vi "UTILITY Add Newfi Data To List.vi"(6 "Use Default Headers Main":bool, 8 "Error In":errorcluster, 10 "Full Data":string[][](array[string]), 11 "New Header Save Array":T1[](array[typedef])) -> (0 "Error Out":errorcluster, 2 "Data":string[][](array[string]), 3 "Save Data":string[][](array[string]))   [LabVIEW 2016]
uses:
  Washer DOE/Type Definitions/DOE Data Save Modifier.ctl
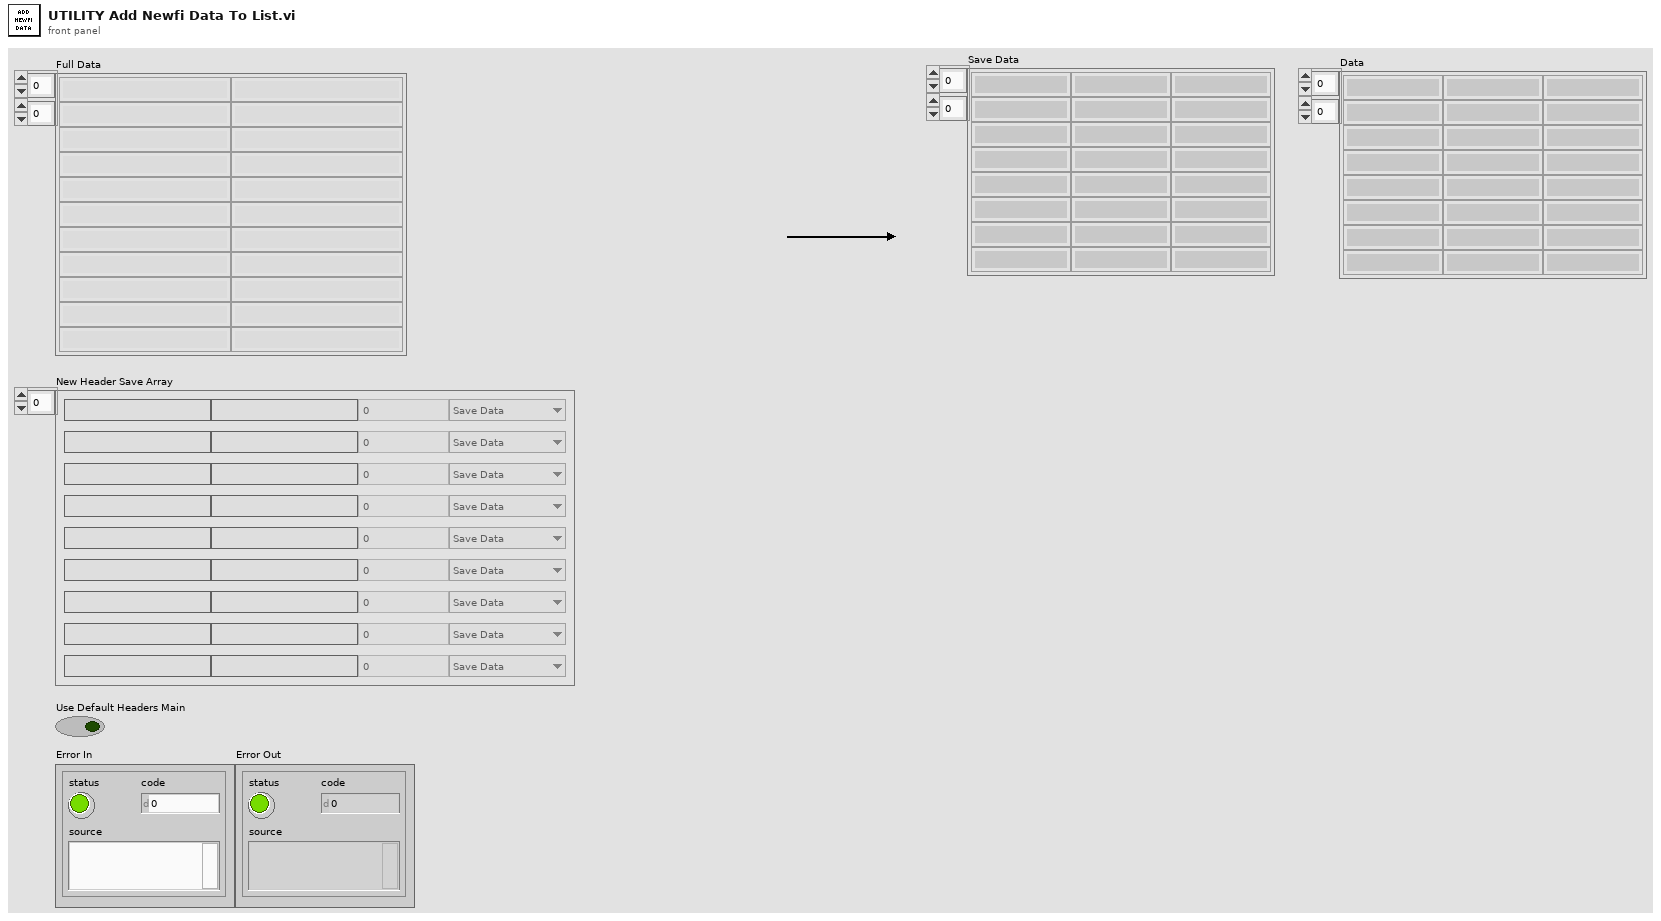
[diagram p1: front panel]
types:
  T1 = typedef "DOE Data Save Modifier.ctl" = cluster{"Name":string, "Title":string, "Save Status":enum16{"Save Data", "Don't Save Data"}, "Group":u8, "Field":u8}
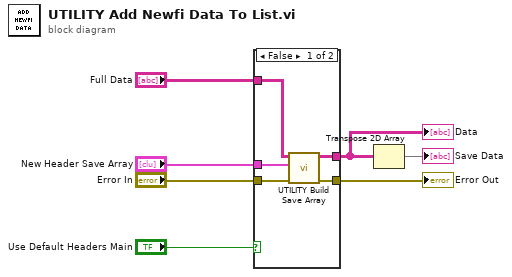
[diagram p0: block diagram]
diagram:
  n1 = case shown="False" "Use Default Headers Main" {
    tunnel: "Full Data" -> [w8 w14]
    tunnel: [w12 w14] -> w7
    tunnel: "New Header Save Array" -> [w11 _]
    tunnel: "Error In" -> [w10 w13]
    tunnel: [w9 w13] -> w2
    frame False {
      n2 = call "UTILITY Build Save Array.vi"("Error In"=w10, "New Header Save Array"=w11, "Full Data Array Out"=w8) -> ("Error Out"=w9:errorcluster, "Selected Data Array Out"=w12:string[][])  [unwired: 7 in]
    }
    frame True {
    }
  }
  "Data" <- w7
  "Error Out" <- w2
  n3 = Transpose 2D Array(2D array=w7) -> (transposed array=→"Save Data":string[][])
